vi "FGV PDF.vi"(6 "Aktion":T3, 10 "Graph":waveform(dbl)(graph) caption="Graph1", 11 "Cluster":T1={"TAB 1"=[["ARN-Test §1065.305", ""], ["Datum und Uhrzeit:", ""], ["Bearbeiter:", ""], ["Messgerät:", "FTIR MKS 2030D EPA ready"], ["Komponente:", ""]], "TAB 2"=[], "TAB 3"=[], "Error"=[]}) -> (2 "Graph":waveform(dbl)(graph) caption="Graph1", 3 "Cluster":T1={"TAB 1"=[["ARN-Test §1065.305", ""], ["Datum und Uhrzeit:", ""], ["Bearbeiter:", ""], ["Messgerät:", "FTIR MKS 2030D EPA ready"], ["Komponente:", ""]], "TAB 2"=[], "TAB 3"=[], "Error"=[]})   [LabVIEW 2020, in "EPA 1065.lvlib" / "ARN Test 1065-305.lvlib"]
uses:
  ARN Test 1065-305.lvlib
  Aktion FGV Protokoll.ctl
  Cluster PDF.ctl
  Visualisierungs Elemente/String - Ausgabefeld.ctl
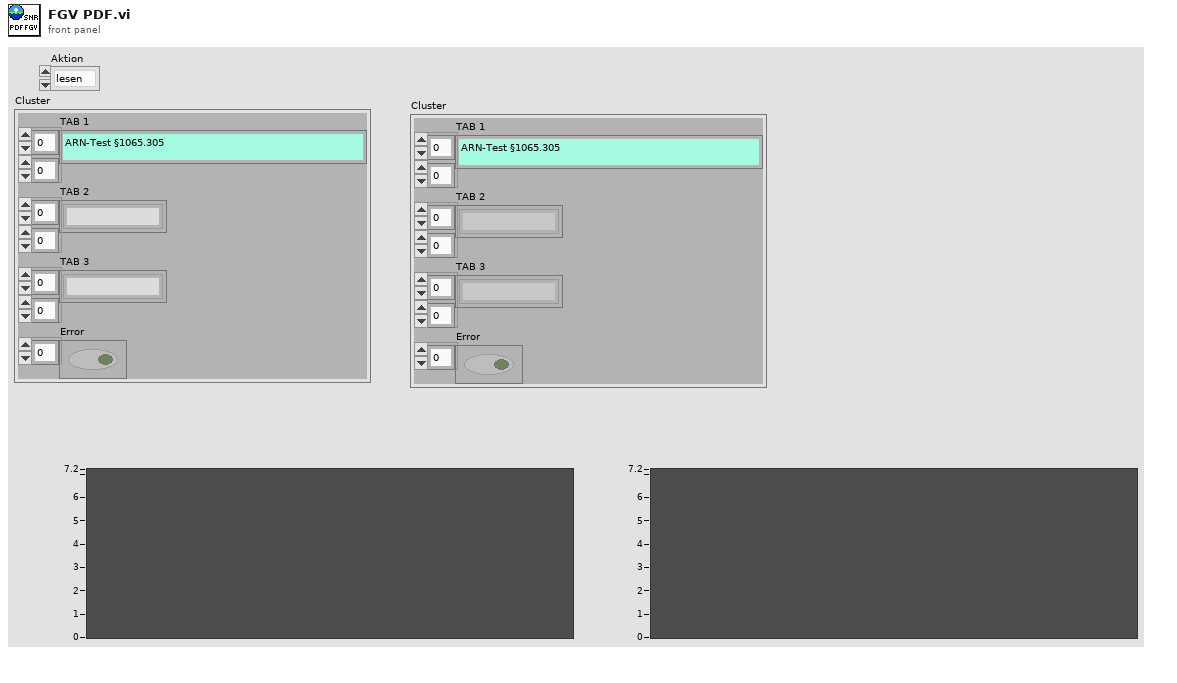
[diagram p1: front panel]
types:
  T1 = typedef "EPA 1065.lvlib/ARN Test 1065-305.lvlib/Cluster PDF.ctl" = cluster{"TAB 1":T2[][], "TAB 2":string[][], "TAB 3":string[][], "Error":bool[]}
  T2 = typedef "String - Ausgabefeld.ctl" = string
  T3 = typedef "EPA 1065.lvlib/ARN Test 1065-305.lvlib/Aktion FGV Protokoll.ctl" = enum16{"lesen", "schreiben", "Graph"}
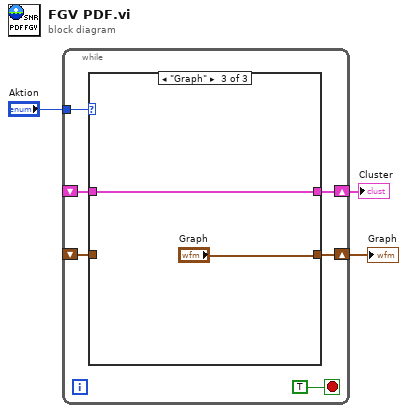
[diagram p0: block diagram]
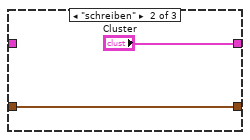
[diagram p3: hidden frame]
diagram:
  n1 = while {
    tunnel: "Aktion" -> [w8]
    shift-right: [w7] -> w2
    shift-left: _ -> [w6]
    shift-right: [w5] -> w1
    shift-left: _ -> [w4]
    stop <- TRUE stop-if-true
    n2 = case shown="\"Graph\"" w8 {
      tunnel: [w11 "Cluster" w15] -> w7
      tunnel: w6 -> [w11 _ w15]
      tunnel: [w10 w12 "Graph"] -> w5
      tunnel: w4 -> [w10 w12 _]
      frame "lesen", Default {
      }
      frame "schreiben" {
      }
      frame "Graph" {
      }
    }
  }
  "Cluster" <- w2
  "Graph" <- w1
